vi "Continuous Voltage Acquisition and Logging.vi"() -> ()   [LabVIEW 2018]
doc: "This example demonstrates how to continuously acquire buffered voltage measurements using a DAQmx device.\n\nFor instructions on how to connect your signals to the DAQ device, refer to your device documentation."
uses:
  <vilib>/Utility/error.llb/DialogType.ctl
  <vilib>/DAQmx/read.llb/DAQmx Read (Analog DBL 1Chan 1Samp).vi
  <vilib>/DAQmx/create/channels.llb/DAQmx Create Channel (AI-Voltage-Basic).vi
  <vilib>/DAQmx/configure/timing.llb/DAQmx Timing (Sample Clock).vi
  <vilib>/DAQmx/configure/task.llb/DAQmx Configure Logging (TDMS).vi
  <vilib>/DAQmx/miscellaneous.llb/DAQmx Fill In Error Info.vi
  <vilib>/Utility/file.llb/Write To Spreadsheet File (string).vi
  <vilib>/Utility/file.llb/Write To Spreadsheet File (DBL).vi
  <resource>/objmgr/daqmx.rc
panel:
  in  "Excel File Name":string caption="add .xls for excel or .tdms, etc"
  out "Log Preview":dbl[][](array[numeric])
  out "Snapshot":dbl(graph)
  out "Amplitude vs Time":cluster{"X":dbl[], "Y":dbl[]}[](graph)
  in  "Enable Excel Log":bool caption="Log Data"
  in  "Stop":bool
  in  "Number of Samples":i32=100
  in  "Sample Rate":dbl=1000.0
  in  "Terminal Configuration":i32(ring)=-1 items=["default"=-1, "RSE"=10083, "NRSE"=10078, "Differential"=10106, "Pseudodifferential"=12529]
  in  "Max Voltage":dbl=5.0
  in  "Min Voltage":dbl=-5.0
  in  "Physical Channel":tag="cDAQ1Mod1/ai0"
  out "Actual Sample Rate":dbl=1000.0 format="%0.2f"
  in  "Acquisition Name":string
  in  "TDMS File Path":path
  in  "Logging Mode":i32(ring)=10231 items=["Off"=10231, "Log and Read"=15842]
  # "Channel Settings"
  # "Timing Settings"
  # "Logging Settings"
  # "Acquired Data"
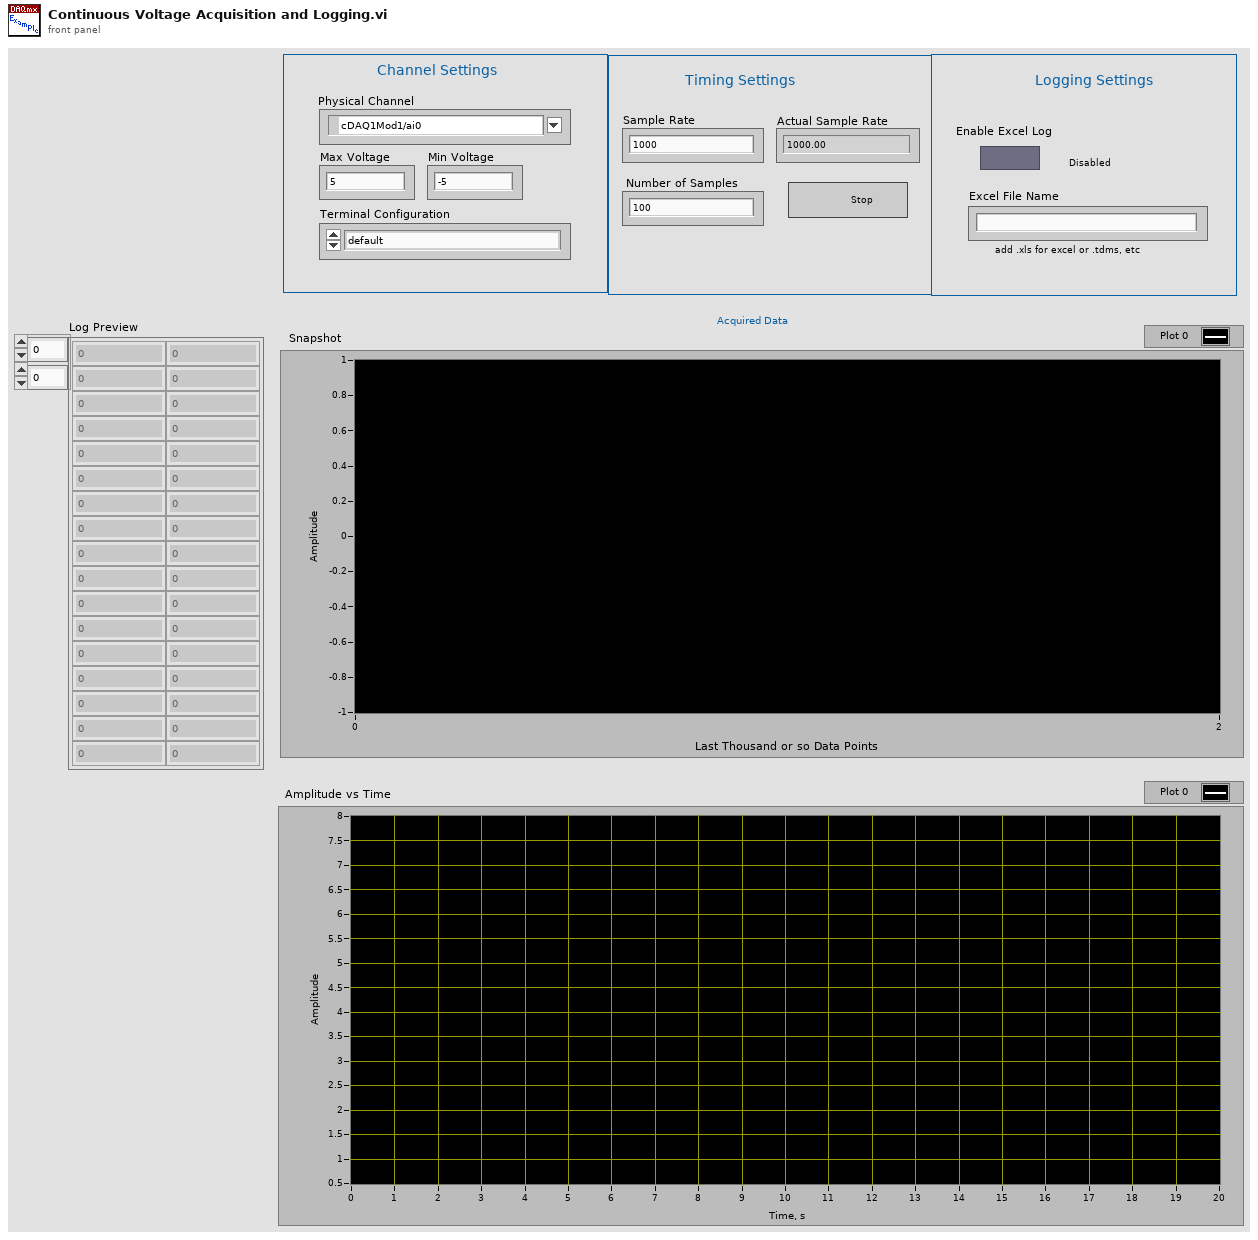
[diagram p1: front panel]
types:
  T1 = typedef "DialogType.ctl" = u16
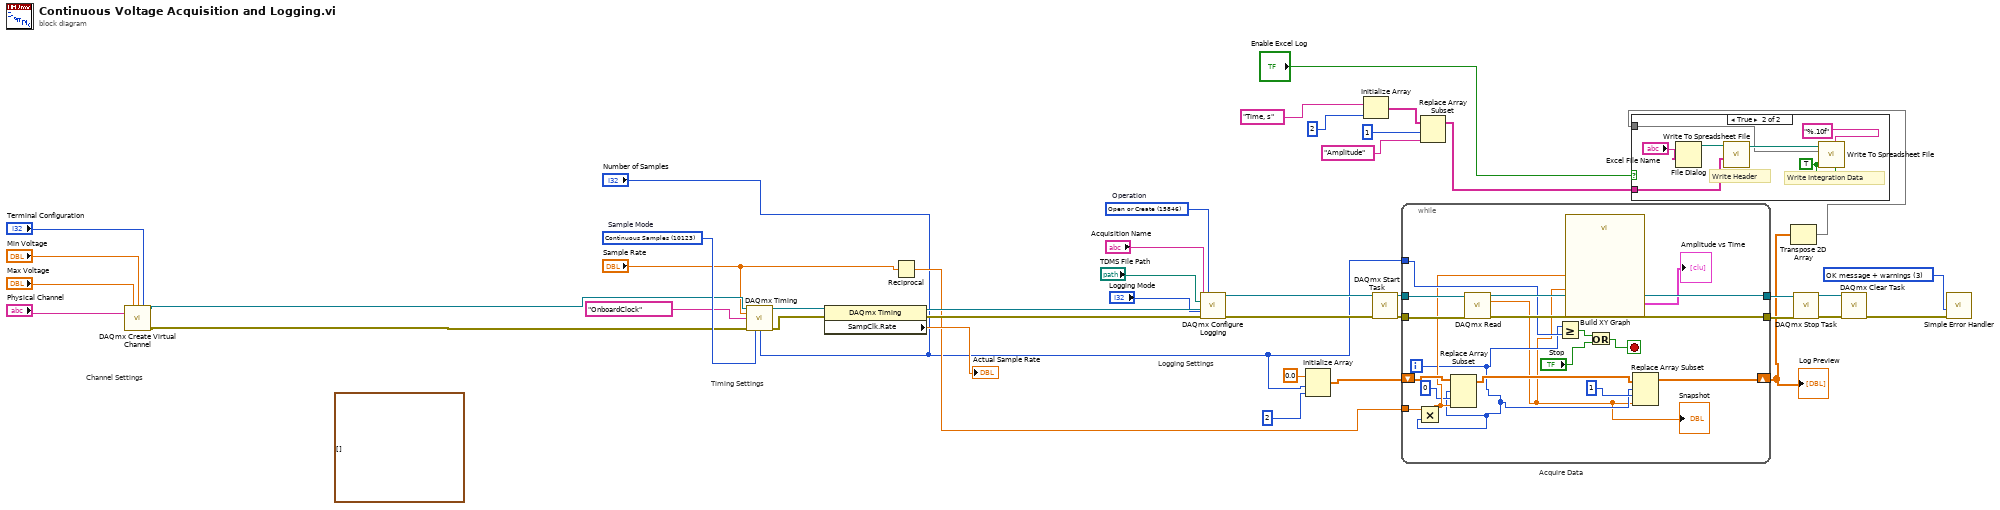
[diagram p0: block diagram]
diagram:
  (unwired) waveform(dbl)[][] [] ("History Data")
  w26 = T1 3 items=["no dialog", "OK message", "continue or stop message", "OK message + warnings", "continue/stop + warnings"] ("type of dialog (OK msg:1)")
  w3 = 15846 items=["Open"=10437, "Open or Create"=15846, "Create or Replace"=15847, "Create"=15848]  # Operation
  w40 = 10123 items=["Finite Samples"=10178, "Continuous Samples"=10123, "Hardware Timed Single Point"=12522]  # Sample Mode
  # "Acquire Data"
  # "Timing Settings"
  # "Channel Settings"
  # "Logging Settings"
  n1 = call-poly <vilib>:"DAQmx Create Virtual Channel.vi"("maximum value"="Max Voltage", "minimum value"="Min Voltage", "input terminal configuration"="Terminal Configuration", "physical channels"="Physical Channel") -> ("task out"=w18:refnum<k21>, "error out"=w1:errorcluster)  [unwired: 10 in]
  n2 = call-poly <vilib>:"DAQmx Timing.vi"("task/channels in"=w18, "sample mode"=w40, "samples per channel"="Number of Samples", "rate"="Sample Rate", "source"=tag "OnboardClock" ("Sample Clock Source"), "error in"=w1) -> ("task out"=w42:refnum<k21>, "error out"=w41:errorcluster)  [unwired: 8 in]
  n3 = property class="DAQmx Timing"(reference=w42, error in=w41) -> (reference out=w39:refnum<k21>, error out=w38:errorcluster, "SampClk.Rate"=→"Actual Sample Rate":dbl)
  n4 = Reciprocal(x="Sample Rate") -> (1/x=w4:dbl)
  n5 = call-poly <vilib>:"DAQmx Configure Logging.vi"("task/channels in"=w39, "operation"=w3, "file path"="TDMS File Path", "group name"="Acquisition Name", "logging mode"="Logging Mode", "error in"=w38) -> ("task out"=w25:refnum<k21>, "error out"=w24:errorcluster)  [unwired: 8 in]
  n6 = Initialize Array(0.0 ("element"), "Number of Samples", 2) -> (w8:dbl[][])
  n7 = Initialize Array("Time, s" ("string"), 2) -> (w12:string[])
  n8 = call <vilib>:"DAQmx Start Task.vi"("task/channels in"=w25, "error in"=w24) -> ("task out"=w37:refnum<k21>, "error out"=w36:errorcluster)  [unwired: 12 in]
  n9 = while {
    tunnel: w37 -> [w60]
    tunnel: w36 -> [w59]
    tunnel: [w58] -> w30
    tunnel: [w57] -> w29
    tunnel: "Number of Samples" -> [w56]
    shift-right: [w44] -> w7
    shift-left: w8 -> [w52]
    tunnel: w4 -> [w50]
    i -> [w45]
    stop <- w53 stop-if-true
    n10 = Multiply(x=w50, y=w45) -> (x*y=w49:dbl)
    n11 = Replace Array Subset(array=w52, new element=w49, index (row)=w45, index (col)=0) -> (w51:dbl[][])
    n12 = call-poly <vilib>:"DAQmx Read.vi"("task/channels in"=w60, "error in"=w59) -> ("task out"=w58:refnum<k21>, "data"=w43:dbl, "error out"=w57:errorcluster)  [unwired: 11 in]
    "Snapshot" <- w43
    n13 = Greater Or Equal?(x=w45, y=w56) -> (x >= y?=w55:bool)
    n14 = call "Build XY Graph"("Y Input"=w43, "X Input"=w49) -> ("XY Graph"=→"Amplitude vs Time":cluster{"X":dbl[], "Y":dbl[]}[])  [unwired: 8 in, 1 out]
    n15 = Or(x=w55, y="Stop") -> (x .or. y?=w53:bool)
    n16 = Replace Array Subset(array=w51, new element=w43, index (row)=w45, index (col)=1) -> (w44:dbl[][])
  }
  "Log Preview" <- w7
  n17 = Replace Array Subset(array=w12, new element="Amplitude" ("string"), index=1) -> (w11:string[])
  n18 = Transpose 2D Array(2D array=w7) -> (transposed array=w6:dbl[][])
  n19 = case shown="True" "Enable Excel Log" {
    tunnel: w6 -> [_ w63]
    tunnel: w11 -> [_ w65]
    frame False {
    }
    frame True {
      w64 = TRUE ("append to file? (new file:F)")
      # "Write Integration Data"
      # "Write Header"
      n20 = File Dialog(9:"Excel File Name") -> (3:w67:path)  [unwired: 1 in, 8 out]
      n21 = call-poly <vilib>:"Write To Spreadsheet File.vi"("1D data"=w65, "file path (dialog if empty)"=w67) -> ("new file path (Not A Path if cancelled)"=w66:path)  [unwired: 4 in, 2 out]
      n22 = call-poly <vilib>:"Write To Spreadsheet File.vi"("transpose? (no:F)"=w64, "format (%.3f)"="%.10f" ("string"), "append to file? (new file:F)"=w64, "2D data"=w63, "file path (dialog if empty)"=w66) -> ()  [unwired: 1 in, 3 out]
    }
  }
  n23 = call <vilib>:"DAQmx Stop Task.vi"("task/channels in"=w30, "error in"=w29) -> ("task out"=w27:refnum<k21>, "error out"=w28:errorcluster)  [unwired: 12 in]
  n24 = call <vilib>:"DAQmx Clear Task.vi"("task in"=w27, "error in"=w28) -> ("error out"=w35:errorcluster)  [unwired: 13 in]
  n25 = call <vilib>:"Simple Error Handler.vi"("type of dialog (OK msg:1)"=w26, "error in (no error)"=w35) -> ()  [unwired: 3 in, 5 out]
